vi "FinalSurvey.vi"(8 "Working Directory to Python scripts":path=path "C:/Users/sciollalab/Desktop/Todd/vi-python", 9 "Folder to save images":path=path "C:/Users/sciollalab/Desktop/Todd/vi-python/histos", 10 "Ideal placement csv path":path=path "C:/Users/sciollalab/Desktop/Todd/vi-python/Stave8Ideals.csv", 11 "Survey csv path":path=path "C:/Users/sciollalab/Desktop/Todd/vi-python/Stave8Survey.csv") -> (1 "Y-histo":T1(plugin-control), 2 "X-histo":T1(plugin-control), 3 "Python standard error":string)   [LabVIEW 2016]
panel:
  out "Y histo path":string
  out "X histo path":string
  in  "Tab Control":enum32{"Page 1", "Page 2"}(tab)
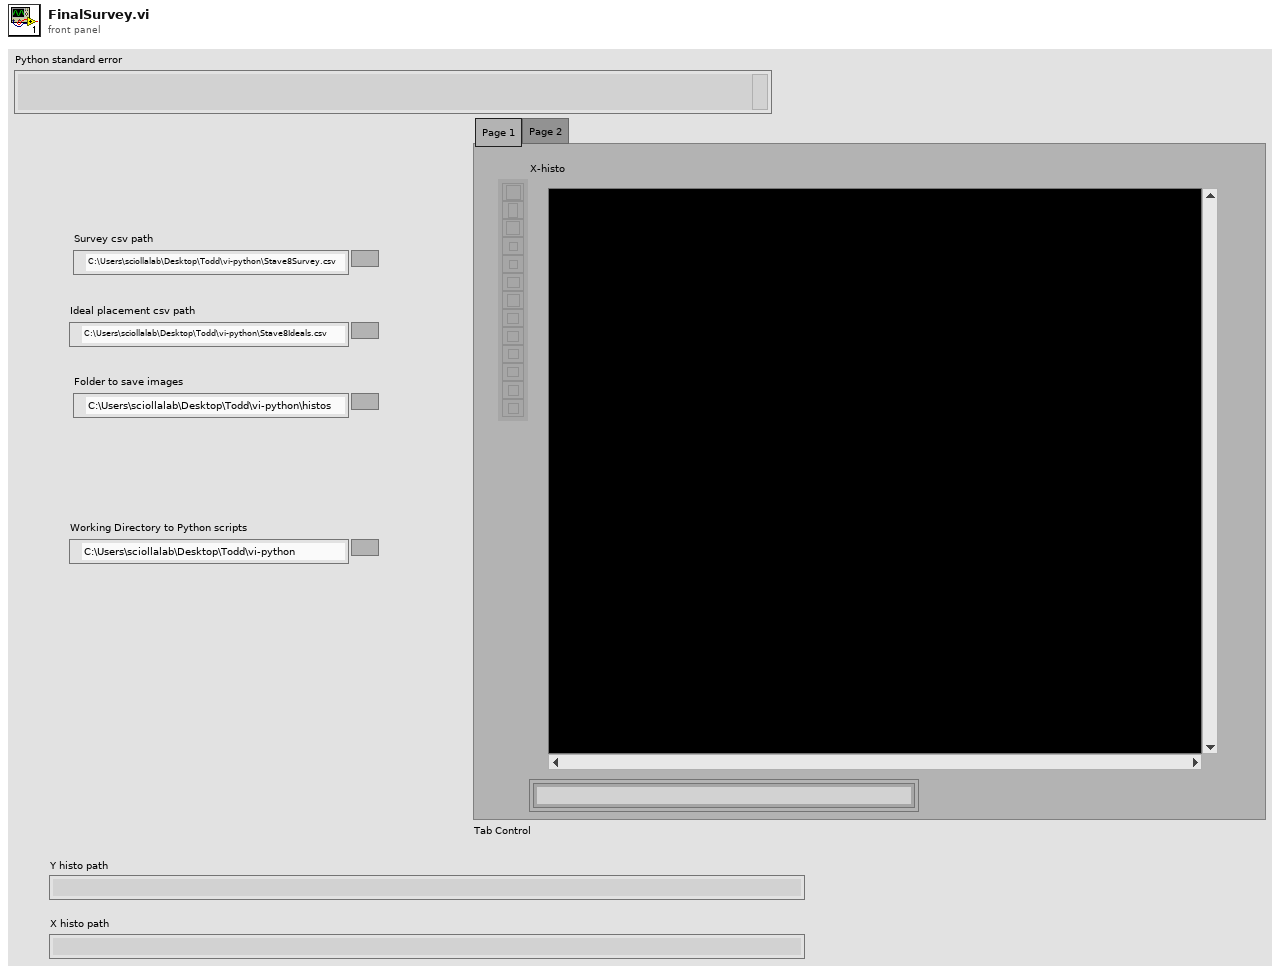
[diagram p1: front panel]
types:
  T1 = typedef "IMAQ Image.ctl" = refnum<image>
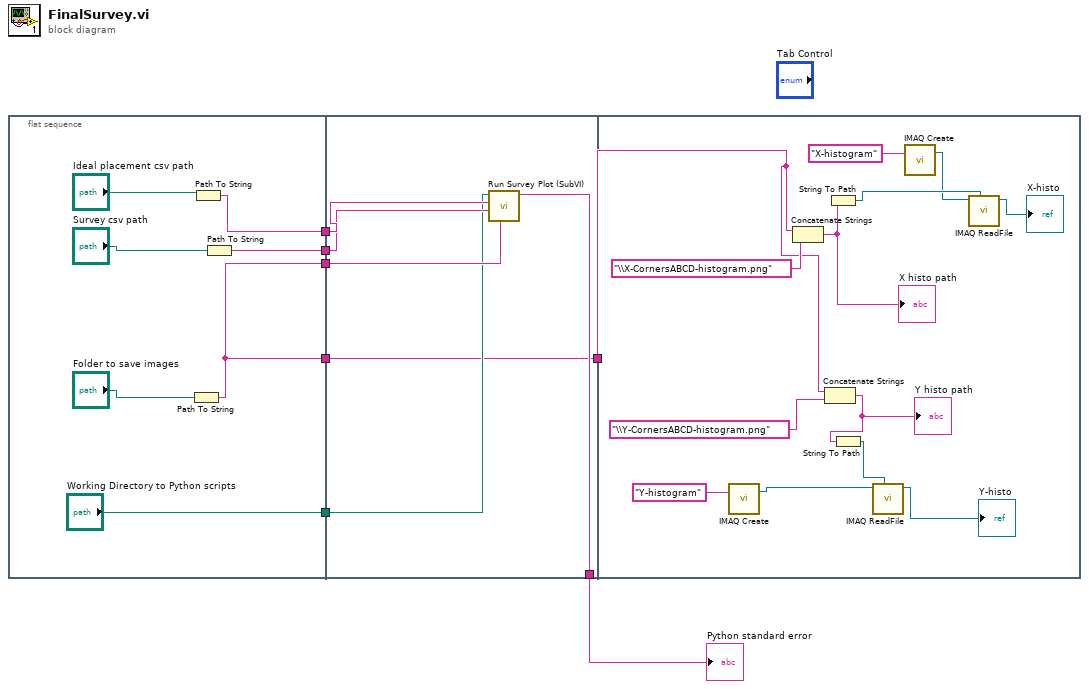
[diagram p0: block diagram]
diagram:
  n1 = flat-sequence {
    tunnel: [w11] -> w7
    tunnel: [w10] -> w6
    tunnel: [w8] -> w5
    tunnel: ["Working Directory to Python scripts"] -> w4
    tunnel: [w8] -> w1
    tunnel: w7 -> [w20]
    tunnel: w6 -> [w19]
    tunnel: w5 -> [w18]
    tunnel: w4 -> [w17]
    tunnel: [w16] -> w3
    tunnel: [w15] -> w2
    tunnel: w1 -> [w15]
    tunnel: w2 -> [w31]
    frame #0 {
      n2 = Path To String(path="Folder to save images") -> (string=w8:string)
      n3 = Path To String(path="Ideal placement csv path") -> (string=w11:string)
      n4 = Path To String(path="Survey csv path") -> (string=w10:string)
    }
    frame #1 {
      n5 = call "Run Survey Plot (SubVI).vi"("Folder to Save"=w18, "Survey csv"=w19, "Ideal csv"=w20, "Working Directory to Python scripts"=w17) -> ("standard error"=w16:string)  [unwired: 7 in]
    }
    frame #2 {
      n6 = call "IMAQ Create"("Image Name"="Y-histogram") -> ("New Image"=w25:T1)  [unwired: 4 in, 1 out]
      n7 = Concatenate Strings(w31, "\\X-CornersABCD-histogram.png") -> (w32:string)
      "X histo path" <- w32
      n8 = Concatenate Strings(w31, "\\Y-CornersABCD-histogram.png") -> (w29:string)
      "Y histo path" <- w29
      n9 = String To Path(string=w32) -> (path=w23:path)
      n10 = String To Path(string=w29) -> (path=w28:path)
      n11 = call "IMAQ ReadFile"("File Path"=w28, "Image"=w25) -> ("Image Out"=→"Y-histo":T1)  [unwired: 5 in, 4 out]
      n12 = call "IMAQ Create"("Image Name"="X-histogram") -> ("New Image"=w22:T1)  [unwired: 4 in, 1 out]
      n13 = call "IMAQ ReadFile"("File Path"=w23, "Image"=w22) -> ("Image Out"=→"X-histo":T1)  [unwired: 5 in, 4 out]
    }
  }
  "Python standard error" <- w3
